vi "FTW-TransferClient-InitializeEvents.vi"(11 "error in":errorcluster) -> (4 "Transfer Begin Timestamp":u32 format="%06dmsec", 6 "Transfer Complete":refnum<user-event>, 8 "Transfer Progress":refnum<user-event>, 10 "Transfer Events":refnum<event-registration>, 15 "error out":errorcluster)   [LabVIEW 2013, in "FTW-TransferClient.lvclass"]
uses:
  FTW-TransferClient.lvclass
  FTW-TransferClient-TransferProgress.ctl
  FTW-TransferClient-TransferStatus.ctl
panel:
  # "Inputs"
  # "Outputs"
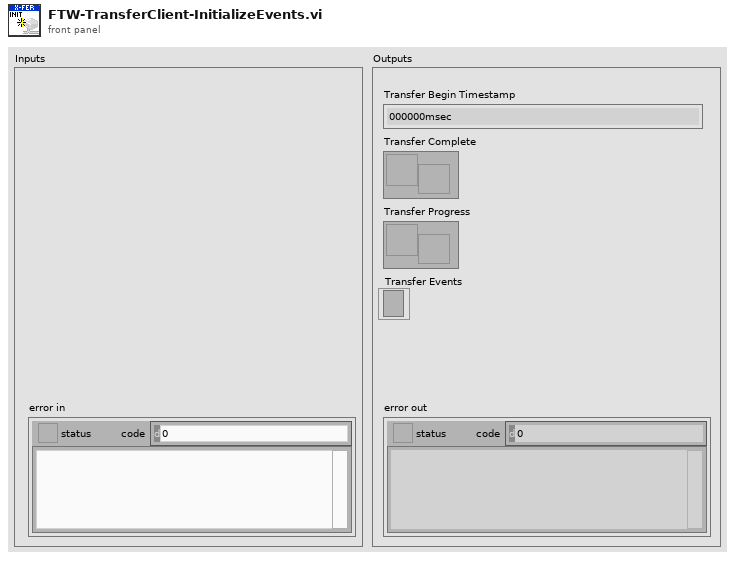
[diagram p1: front panel]
types:
  T1 = typedef "FTW-TransferClient-TransferStatus.ctl" = cluster{"Remote URI":string, "Local Filepath":path, "Cancelled?":bool, "Error?":bool, "Error Message":string, "Time Elapsed":u32}
  T2 = typedef "FTW-TransferClient-TransferProgress.ctl" = cluster{"Remote URI":string, "Local Filepath":path, "Total Bytes":i64, "Transferred Bytes":i64, "Percent Complete":dbl, "Current Rate":dbl, "Time Elapsed":u32, "Est. Time Remaining":u32}
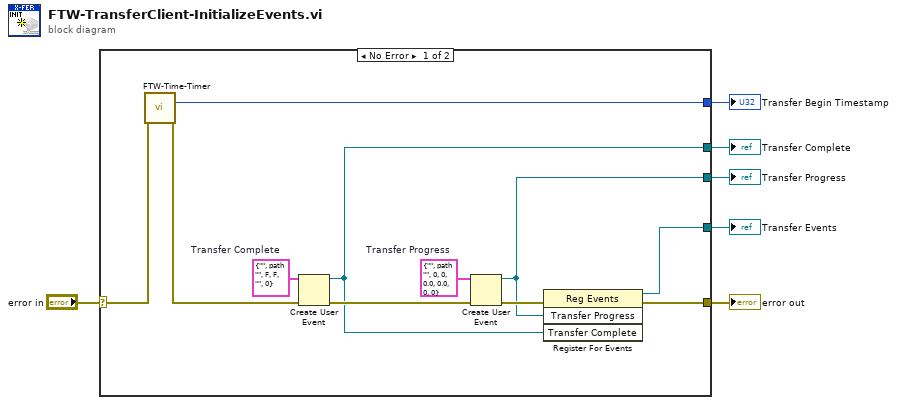
[diagram p0: block diagram]
diagram:
  n1 = case shown="No Error" "error in" {
    selector: "error in" -> [w15 w18]
    tunnel: [w13 w18] -> w6
    tunnel: [w9 _] -> w4
    tunnel: [w8 _] -> w3
    tunnel: [w14 _] -> w2
    tunnel: [w7 _] -> w1
    frame No Error {
      w16 = T1 {"Remote URI"="", "Local Filepath"=path "", "Cancelled?"=FALSE, "Error?"=FALSE, "Error Message"="", "Time Elapsed"=0}  # Transfer Complete
      w17 = T2 {"Remote URI"="", "Local Filepath"=path "", "Total Bytes"=0, "Transferred Bytes"=0, "Percent Complete"=0.0, "Current Rate"=0.0, "Time Elapsed"=0, "Est. Time Remaining"=0}  # Transfer Progress
      n2 = call "FTW-Time-Timer.vi"("error in"=w15) -> ("Elapsed Time"=w14:u32, "error out"=w12:errorcluster)  [unwired: 12 in, 1 out]
      n3 = Create User Event(user event datatype=w16, error in=w12) -> (user event=w8:refnum<user-event>, error out=w11:errorcluster)
      n4 = Create User Event(user event datatype=w17, error in=w11) -> (user event=w9:refnum<user-event>, error out=w10:errorcluster)
      n5 = register-events(error in=w10, w9, w8) -> (reference out=w7:refnum<event-registration>, error out=w13:errorcluster)  [unwired: 1 in]
    }
    frame Error {
    }
  }
  "error out" <- w6
  "Transfer Progress" <- w4
  "Transfer Complete" <- w3
  "Transfer Begin Timestamp" <- w2
  "Transfer Events" <- w1
